vi "Write Serial Number.vi"(10 "Serial Number":string, 11 "Instrument in":refnum<class "Instrument.lvclass">) -> (3 "Instrument out":refnum<class "Instrument.lvclass">)   [LabVIEW 2020, in "Instrument.lvclass"]
uses:
  Instrument.lvclass
  Instrument.lvclass/Instrument.ctl
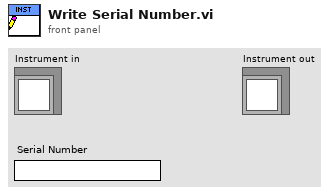
[diagram p1: front panel]
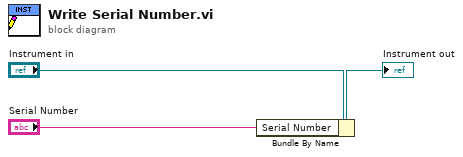
[diagram p0: block diagram]
diagram:
  n1 = Bundle By Name(cluster="Instrument in", "Serial Number"="Serial Number") -> (→"Instrument out":refnum<class "Instrument.lvclass">)
